vi "Download Winding.vi"(8 "error in (no error)":errorcluster, 9 "index":i32, 10 "Array":T1(array[cluster]), 11 "Programing Logic in":refnum<class "Programing Logic.lvclass">) -> (0 "error out":errorcluster, 3 "Programing Logic out":refnum<class "Programing Logic.lvclass">)   [LabVIEW 2014, in "Programing Logic.lvclass"]
uses:
  Programing Logic.lvclass
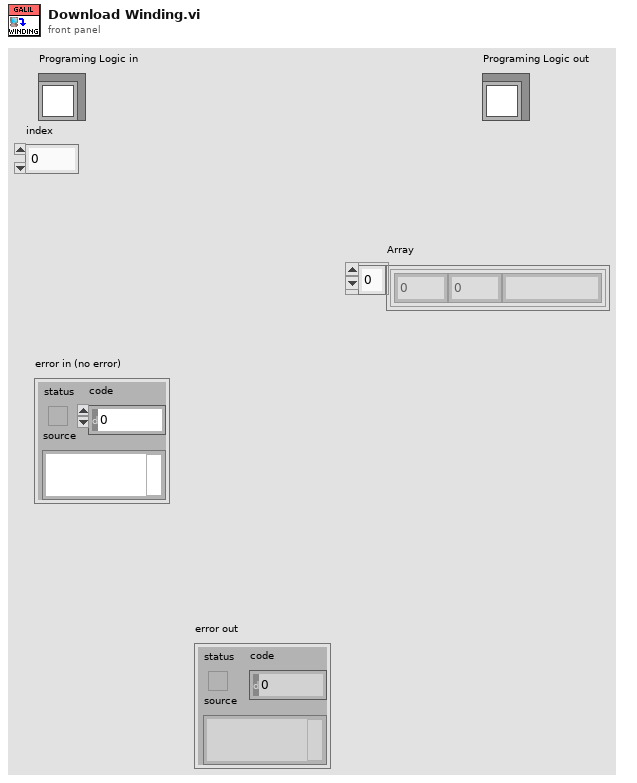
[diagram p1: front panel]
types:
  T1 = cluster{"Numeric":dbl, "Numeric 2":dbl, "String":string}[]
  T2 = cluster{"Numeric":dbl, "Numeric 2":dbl, "String":string}
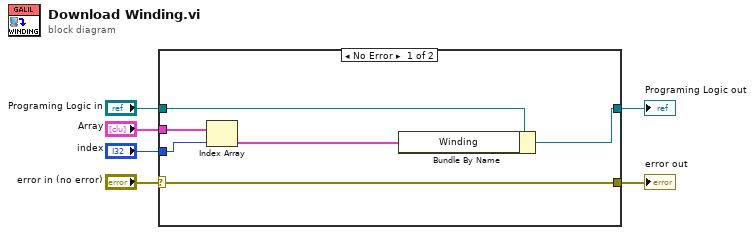
[diagram p0: block diagram]
diagram:
  n1 = case shown="No Error" "error in (no error)" {
    selector: "error in (no error)" -> [w12 w14]
    tunnel: [w12 w14] -> w5
    tunnel: [w10 w13] -> w3
    tunnel: "Programing Logic in" -> [w11 w13]
    tunnel: "Array" -> [w9 _]
    tunnel: "index" -> [w7 _]
    frame No Error {
      n2 = Index Array(array=w9, index=w7) -> (element=w8:T2)
      n3 = Bundle By Name(cluster=w11, "Winding"=w8) -> (w10:refnum<class "Programing Logic.lvclass">)
    }
    frame Error {
    }
  }
  "error out" <- w5
  "Programing Logic out" <- w3
